vi "Agilent E3633 DC PS_driver.vi"(6 "VISA resource in":refnum<visa-resource-name>, 7 "Enable Output (T: Enable)":bool=TRUE, 8 "Error In":errorcluster, 9 "value in":dbl, 10 "agilent E3633 DC PS":T1) -> (0 "Error Out":errorcluster, 1 "I out":dbl, 2 "V out":dbl, 4 "VISA resource name out":refnum<visa-resource-name>)   [LabVIEW 2020]
uses:
  dc ps control.ctl
  <instrlib>/Agilent E363X/Agilent E363X Series.lvlib
panel:
  out "Self-Test Result Message":string
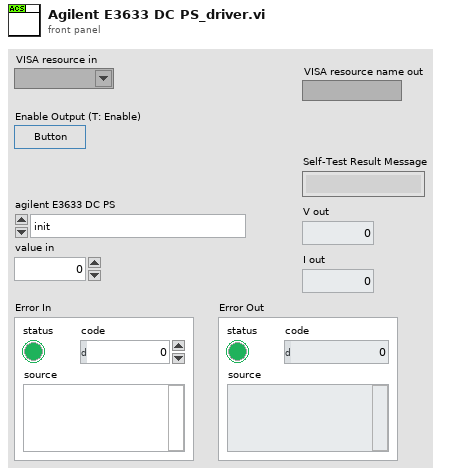
[diagram p1: front panel]
types:
  T1 = typedef "dc ps control.ctl" = enum16{"init", "config output", "config OVP", "config current limit", "output on_off", "read output", "self test", "close"}
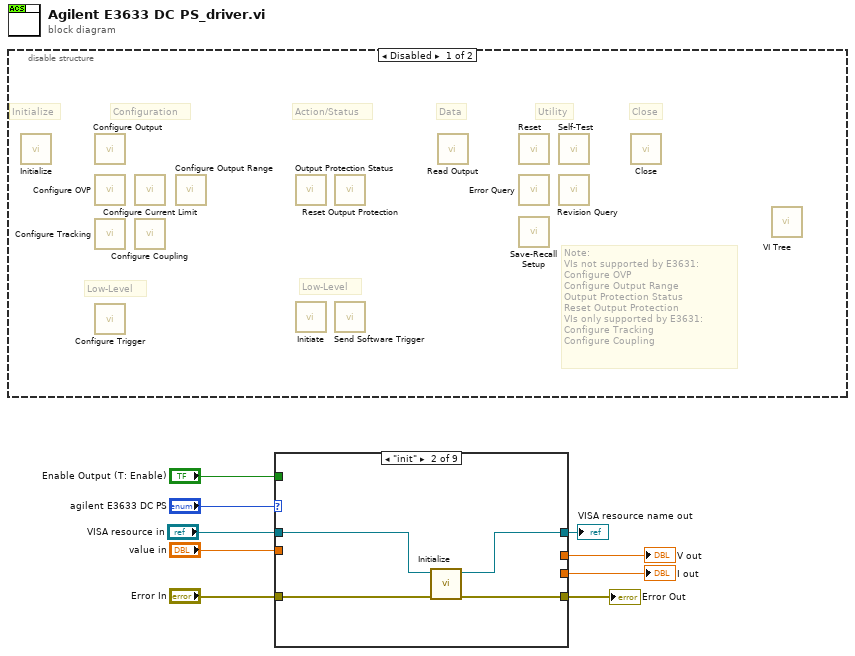
[diagram p0: block diagram]
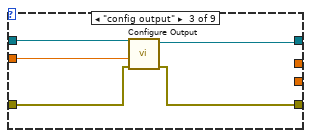
[diagram p3: hidden frame]
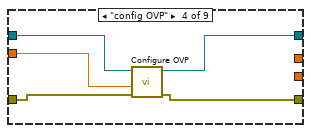
[diagram p4: hidden frame]
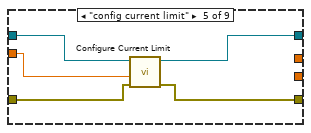
[diagram p5: hidden frame]
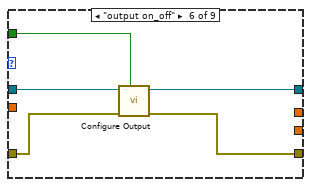
[diagram p6: hidden frame]
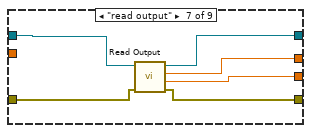
[diagram p7: hidden frame]
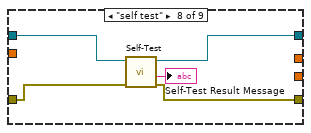
[diagram p8: hidden frame]
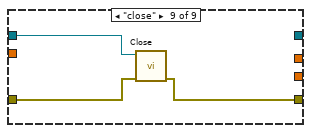
[diagram p9: hidden frame]
diagram:
  n1 = disable-structure shown="Disabled" {
    frame Disabled {
      # "Note:\nVIs not supported by E3631:\nConfigure OVP\nConfigure Output Range\nOutput Protection Status\nReset Output Protection\nVIs only supported by E3631:\nConfigure Tracking\nConfigure Coupling"
      # "Low-Level"
      # "Low-Level"
      # "Configuration"
      # "Utility"
      # "Data"
      # "Action/Status"
      # "Close"
      # "Initialize"
      n2 = call <instrlib>:"Initialize.vi"() -> ()  [unwired: 10 in, 2 out]
      n3 = call <instrlib>:"Configure Output.vi"() -> ()  [unwired: 10 in, 2 out]
      n4 = call <instrlib>:"Configure OVP.vi"() -> ()  [unwired: 10 in, 2 out]
      n5 = call <instrlib>:"Configure Tracking.vi"() -> ()  [unwired: 10 in, 2 out]
      n6 = call <instrlib>:"Configure Trigger.vi"() -> ()  [unwired: 10 in, 2 out]
      n7 = call <instrlib>:"Configure Current Limit.vi"() -> ()  [unwired: 10 in, 2 out]
      n8 = call <instrlib>:"Configure Coupling.vi"() -> ()  [unwired: 10 in, 2 out]
      n9 = call <instrlib>:"Configure Output Range.vi"() -> ()  [unwired: 10 in, 2 out]
      n10 = call <instrlib>:"Output Protection Status.vi"() -> ()  [unwired: 8 in, 4 out]
      n11 = call <instrlib>:"Initiate.vi"() -> ()  [unwired: 10 in, 2 out]
      n12 = call <instrlib>:"Reset Output Protection.vi"() -> ()  [unwired: 10 in, 2 out]
      n13 = call <instrlib>:"Send Software Trigger.vi"() -> ()  [unwired: 10 in, 2 out]
      n14 = call <instrlib>:"Read Output.vi"() -> ()  [unwired: 8 in, 4 out]
      n15 = call <instrlib>:"Reset.vi"() -> ()  [unwired: 10 in, 2 out]
      n16 = call <instrlib>:"Error Query.vi"() -> ()  [unwired: 8 in, 4 out]
      n17 = call <instrlib>:"Save-Recall Setup.vi"() -> ()  [unwired: 10 in, 2 out]
      n18 = call <instrlib>:"Self-Test.vi"() -> ()  [unwired: 8 in, 4 out]
      n19 = call <instrlib>:"Revision Query.vi"() -> ()  [unwired: 8 in, 4 out]
      n20 = call <instrlib>:"Close.vi"() -> ()  [unwired: 11 in, 1 out]
      n21 = call <instrlib>:"VI Tree.vi"() -> ()  [unwired: 12 in]
    }
    frame Enabled {
    }
  }
  n22 = case shown="\"init\"" "agilent E3633 DC PS" {
    tunnel: "Error In" -> [w11 w15 w19 w22 w30 w32 w39 w43 w48]
    tunnel: [w11 w14 w18 w21 w29 w31 w38 w42 w47] -> w7
    tunnel: [w10 w13 w17 w24 w27 w34 w40 w45 _] -> w1
    tunnel: "VISA resource in" -> [w10 w12 w20 w25 w28 w35 w41 w46 w49]
    tunnel: "value in" -> [_ _ w16 w23 w26 _ _ _ _]
    tunnel: "Enable Output (T: Enable)" -> [_ _ _ _ _ w33 _ _ _]
    tunnel: [_ _ _ _ _ _ w37 _ _] -> w4
    tunnel: [_ _ _ _ _ _ w36 _ _] -> w3
    frame Default {
    }
    frame "init" {
      n23 = call <instrlib>:"Initialize.vi"("error in (no error)"=w15, "VISA resource name"=w12) -> ("error out"=w14:errorcluster, "VISA resource name out"=w13:refnum<visa-resource-name>)  [unwired: 8 in]
    }
    frame "config output" {
      n24 = call <instrlib>:"Configure Output.vi"("error in (no error)"=w19, "Voltage Level (0.0 V)"=w16, "VISA resource name"=w20) -> ("error out"=w18:errorcluster, "VISA resource name out"=w17:refnum<visa-resource-name>)  [unwired: 7 in]
    }
    frame "config OVP" {
      n25 = call <instrlib>:"Configure OVP.vi"("error in (no error)"=w22, "Voltage Limit (0.0 V)"=w23, "VISA resource name"=w25) -> ("error out"=w21:errorcluster, "VISA resource name out"=w24:refnum<visa-resource-name>)  [unwired: 7 in]
    }
    frame "config current limit" {
      n26 = call <instrlib>:"Configure Current Limit.vi"("error in (no error)"=w30, "Current Limit (0.0 A)"=w26, "VISA resource name"=w28) -> ("error out"=w29:errorcluster, "VISA resource name out"=w27:refnum<visa-resource-name>)  [unwired: 7 in]
    }
    frame "output on_off" {
      n27 = call <instrlib>:"Configure Output.vi"("Enable Output (T: Enable)"=w33, "error in (no error)"=w32, "VISA resource name"=w35) -> ("error out"=w31:errorcluster, "VISA resource name out"=w34:refnum<visa-resource-name>)  [unwired: 7 in]
    }
    frame "read output" {
      n28 = call <instrlib>:"Read Output.vi"("error in (no error)"=w39, "VISA resource name"=w41) -> ("error out"=w38:errorcluster, "Actual Current Level (A)"=w36:dbl, "Actual Voltage Level (V)"=w37:dbl, "VISA resource name out"=w40:refnum<visa-resource-name>)  [unwired: 6 in]
    }
    frame "self test" {
      n29 = call <instrlib>:"Self-Test.vi"("error in (no error)"=w43, "VISA resource name"=w46) -> ("error out"=w42:errorcluster, "Self-Test Result Message"=→"Self-Test Result Message":string, "VISA resource name out"=w45:refnum<visa-resource-name>)  [unwired: 6 in, 1 out]
    }
    frame "close" {
      n30 = call <instrlib>:"Close.vi"("error in (no error)"=w48, "VISA resource name"=w49) -> ("error out"=w47:errorcluster)  [unwired: 9 in]
    }
  }
  "Error Out" <- w7
  "V out" <- w4
  "I out" <- w3
  "VISA resource name out" <- w1
